vi "first vi.vi"() -> ()   [LabVIEW 2019]
panel:
  in  "OK Button":bool
  in  "Boolean 2":bool
  out "String 2":string
  in  "String":string
  out "Boolean 3":bool
  in  "Boolean":bool
  out "Meter":dbl(knob) scale=0.0..10.0
  in  "Knob":cluster{dbl, dbl}(knob) scale=0.0..1e+23
  in  "Slide":dbl(slide) scale=0.0..10.0
  out "Slide 2":dbl(slide) scale=0.0..10.0
  out "Numeric 2":dbl
  in  "Numeric":dbl
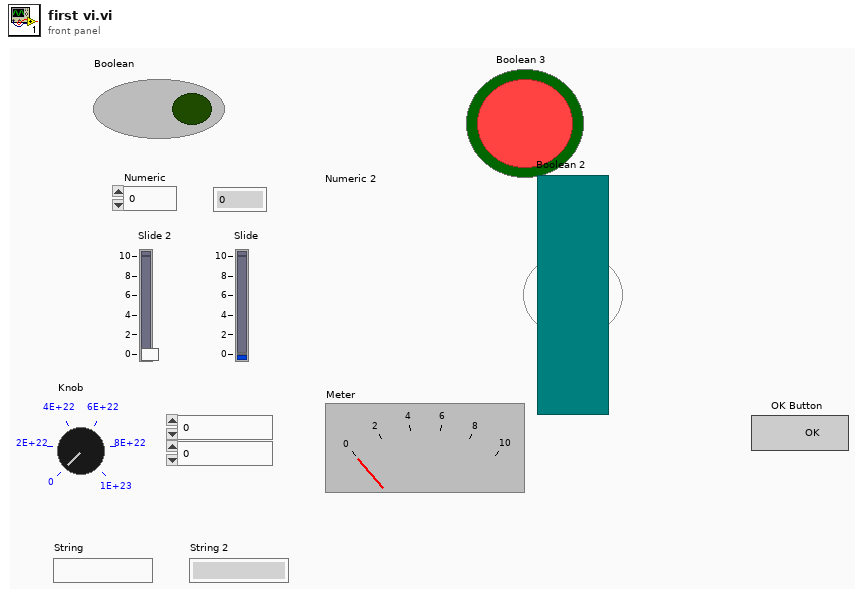
[diagram p1: front panel]
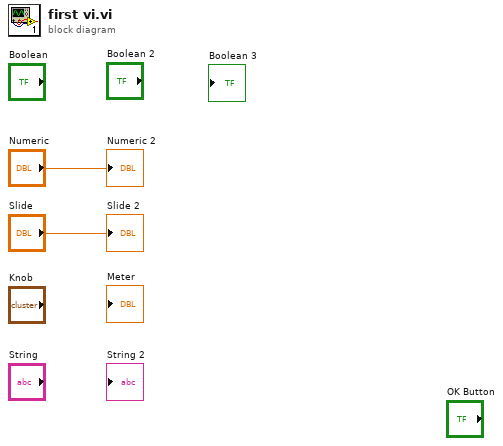
[diagram p0: block diagram]
diagram:
  "Numeric 2" <- "Numeric"
  "Slide 2" <- "Slide"
